vi "MStar Daily產能安排Report.vi"() -> ()   [LabVIEW 2012]
uses:
  <vilib>/Utility/NIReport.llb/NI_report.lvclass
  <vilib>/addons/database/Connection.llb/DB Tools Open Connec (Path).vi
  <vilib>/addons/database/Connection.llb/Conn Execute.vi
  <vilib>/addons/database/Recordset.llb/Rec Fetch Recordset Data (R).vi
  <vilib>/addons/database/Recordset.llb/Rec Destroy - Connection.vi
  <vilib>/Utility/NIReport.llb/Append Text Table to Report (wrap).vi
  <vilib>/addons/database/_DB Variant To Data/Database Variant To Data.xnode
  <vilib>/addons/database/NI_Database_API.lvlib
  <vilib>/Utility/NIReport.llb/Excel/NI_Excel.lvclass
panel:
  out "recordset data":variant[][](array[variant])
  out "appended array":string[](array[string])
  in  "Report Template":path=path "O:/Monitor/Report/MachineArrange.xls"
  out "error out 2":errorcluster
  in  "Table Control":string[][](table)
  out "error out 3":errorcluster
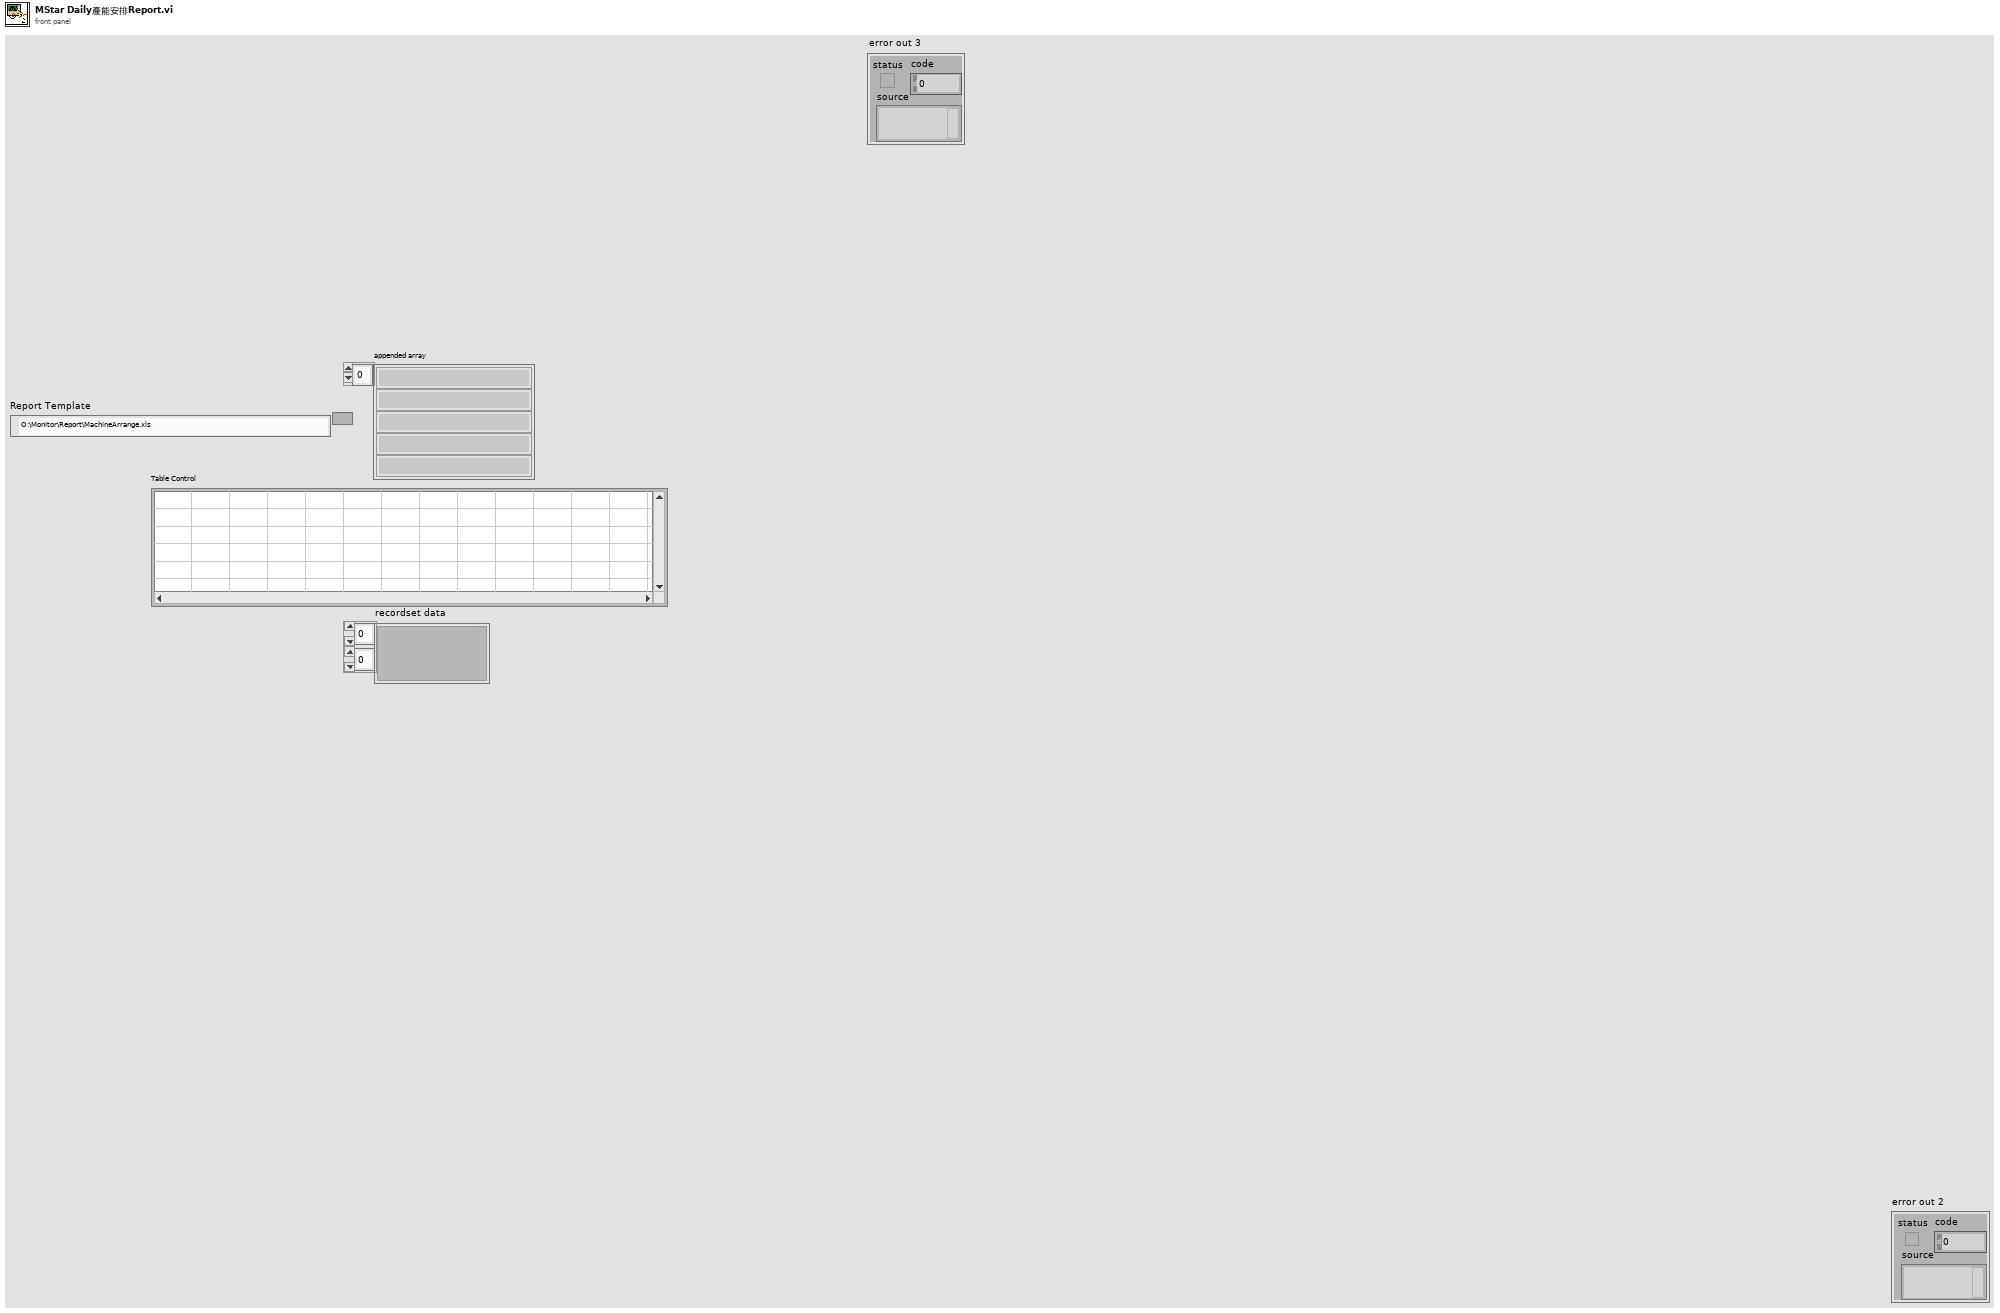
[diagram p1: front panel]
types:
  T1 = typedef "NI_Database_API.lvlib/Conn ObjectReference.ctl" = refnum<k1>
  T2 = typedef "NI_Database_API.lvlib/Rec ObjectReference.ctl" = refnum<k1>
  T3 = enum16{"Standard Report", "HTML", "Word", "Excel"}
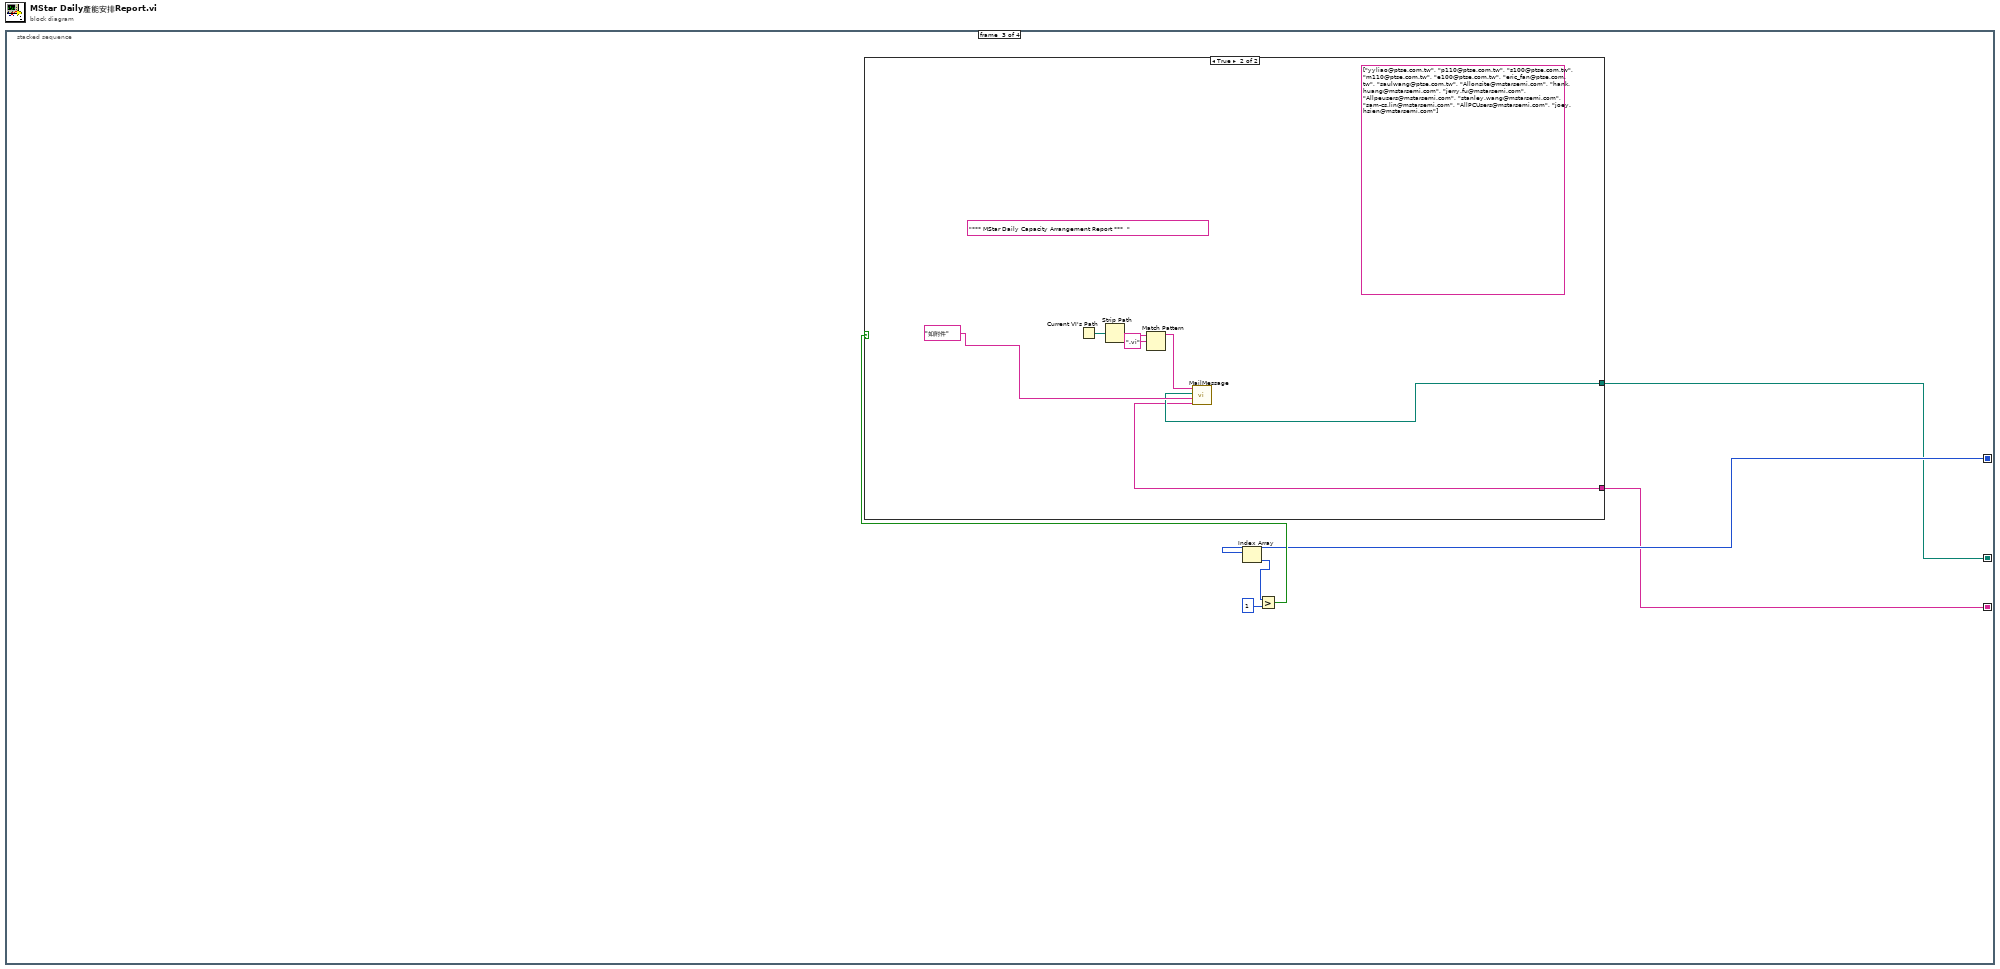
[diagram p0: block diagram]
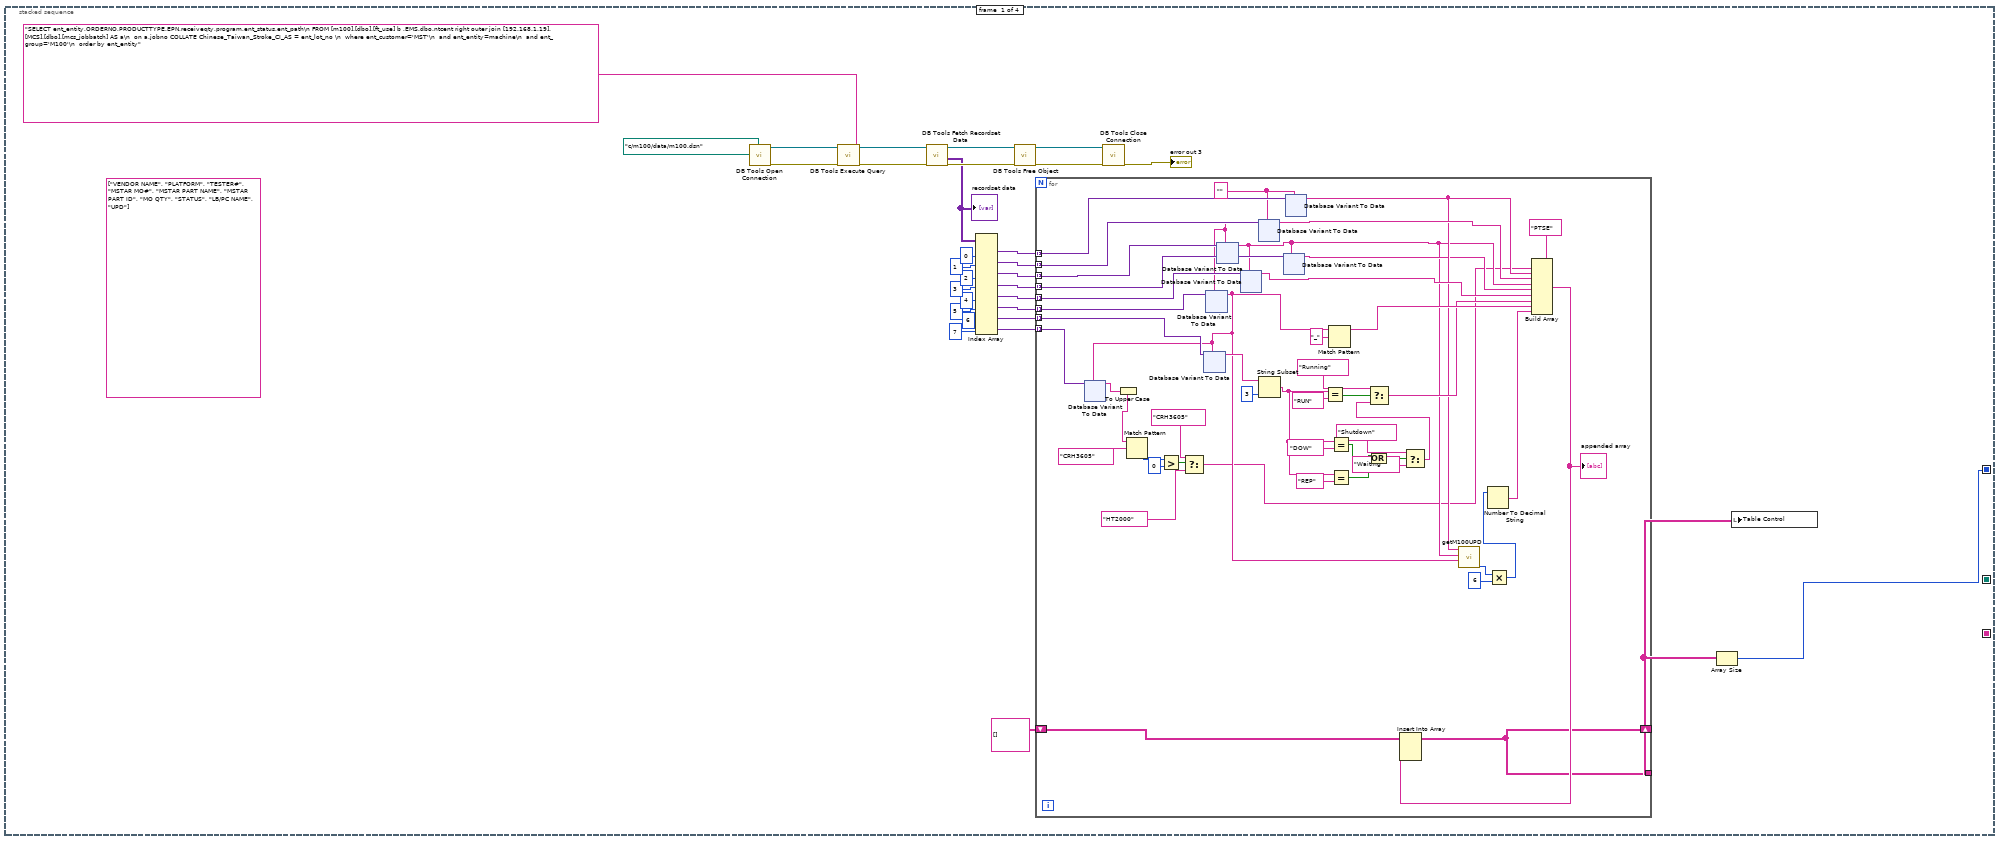
[diagram p2: hidden frame]
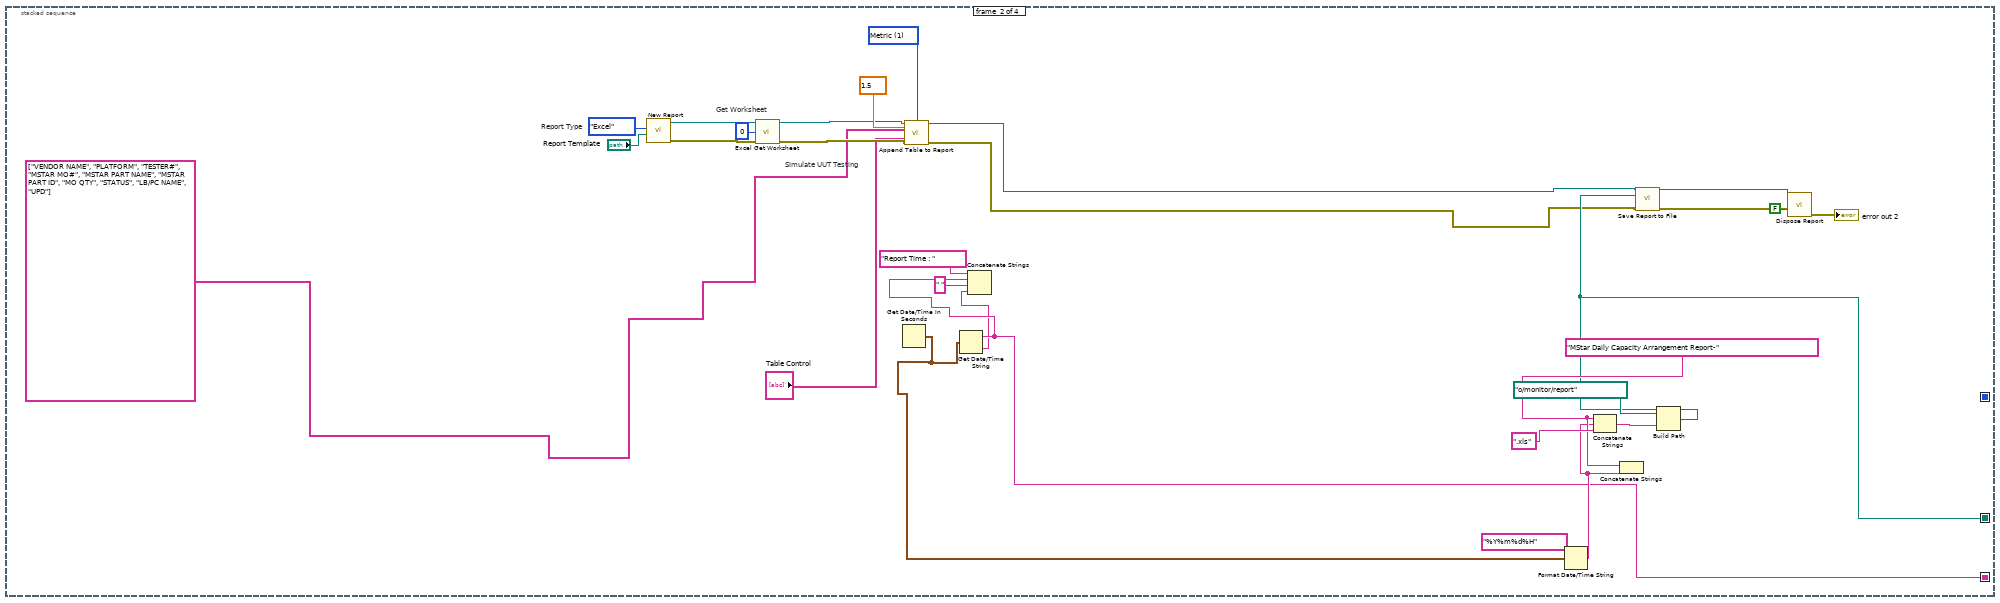
[diagram p3: hidden frame]
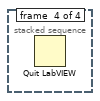
[diagram p5: hidden frame]
diagram:
  n1 = stacked-sequence {
    seq-local: [w5 _ _ _] -> [_ _ w368 _]
    seq-local: [_ w345 _ _] -> [_ _ w367 _]
    seq-local: [_ w342 _ _] -> [_ _ w366 _]
    frame #0 {
      (unwired) string[] ["VENDOR NAME", "PLATFORM", "TESTER#", "MSTAR MO#", "MSTAR PART NAME", "MSTAR PART ID", "MO QTY", "STATUS", "LB/PC NAME", "UPD"] ("row headers")
      n2 = call-poly <vilib>:"DB Tools Open Connection.vi"("connection information"=path "c:/m100/data/m100.dsn") -> ("error out"=w26:errorcluster, "connection reference"=w30:T1)  [unwired: 7 in]
      n3 = call-poly <vilib>:"DB Tools Execute Query.vi"("error in (no error)"=w26, "SQL query"="SELECT ent_entity,ORDERNO,PRODUCTTYPE,EPN,receiveqty,program,ent_status,ent_path\n FROM [m100].[dbo].[ft_use] b ,EMS.dbo.ntcent right outer join [192.168.1.19].[MCS].[dbo].[mcs_jobbatch] AS a\n  on a.jobno COLLATE Chinese_Taiwan_Stroke_CI_AS = ent_lot_no \n  where ent_customer='MST'\n  and ent_entity=machine\n  and ent_group='M100'\n  order by ent_entity", "connection reference"=w30) -> ("error out"=w25:errorcluster, "recordset reference"=w29:T2)  [unwired: 5 in]
      n4 = call-poly <vilib>:"DB Tools Fetch Recordset Data.vi"("error in (no error)"=w25, "recordset reference"=w29) -> ("error out"=w24:errorcluster, "recordset data"=w8:variant[][], "recordset reference out"=w28:T2)  [unwired: 3 in]
      "recordset data" <- w8
      n5 = Index Array(array=w8, index (col) #1=0 ("disabled index (col)"), index (col) #2=1 ("index (col)"), index (col) #3=2 ("index (col)"), index (col) #4=3 ("index (col)"), index (col) #5=4 ("index (col)"), index (col) #6=5 ("index (col)"), index (col) #7=6 ("index (col)"), index (col) #8=7 ("index (col)")) -> (element #1=w15:variant[], element #2=w14:variant[], element #3=w13:variant[], element #4=w12:variant[], element #5=w11:variant[], element #6=w10:variant[], element #7=w3:variant[], element #8=w1:variant[])  [unwired: 8 in]
      n6 = call-poly <vilib>:"DB Tools Free Object.vi"("error in (no error)"=w24, "recordset reference"=w28) -> ("error out"=w23:errorcluster, "connection reference"=w27:T1)  [unwired: 8 in]
      n7 = for {
        tunnel: w15 -> [w80] mode=indexing
        tunnel: w14 -> [w79] mode=indexing
        tunnel: w13 -> [w78] mode=indexing
        tunnel: w12 -> [w77] mode=indexing
        tunnel: w11 -> [w76] mode=indexing
        tunnel: w10 -> [w75] mode=indexing
        tunnel: [w73] -> w6
        shift-right: [w73] -> _
        shift-left: string[][] [] -> [w72]
        tunnel: w3 -> [w66] mode=indexing
        tunnel: w1 -> [w45] mode=indexing
        w70 = ""
        n8 = xnode "Database Variant To Data"("database variant"=w75, "type"=w70) -> ("data"=w44:string)  [unwired: 1 in, 1 out]
        n9 = xnode "Database Variant To Data"("database variant"=w45, "type"=w44) -> ("data"=w36:string)  [unwired: 1 in, 1 out]
        n10 = To Upper Case(1:w36) -> (0:w35:string)
        n11 = Match Pattern(string=w35, regular expression="CRH3605") -> (offset past match=w42:i32)  [unwired: 1 in, 3 out]
        n12 = Greater?(x=w42, y=0) -> (0:w40:bool)
        n13 = Select(t="CRH3605", s=w40, f="HT2000") -> (s? t:f=w37:string)
        n14 = xnode "Database Variant To Data"("database variant"=w66, "type"=w44) -> ("data"=w65:string)  [unwired: 1 in, 1 out]
        n15 = xnode "Database Variant To Data"("database variant"=w78, "type"=w70) -> ("data"=w46:string)  [unwired: 1 in, 1 out]
        n16 = xnode "Database Variant To Data"("database variant"=w76, "type"=w46) -> ("data"=w69:string)  [unwired: 1 in, 1 out]
        n17 = xnode "Database Variant To Data"("database variant"=w79, "type"=w70) -> ("data"=w71:string)  [unwired: 1 in, 1 out]
        n18 = String Subset(string=w65, length (rest)=3 ("length (rest)")) -> (substring=w58:string)  [unwired: 1 in]
        n19 = xnode "Database Variant To Data"("database variant"=w77, "type"=w46) -> ("data"=w48:string)  [unwired: 1 in, 1 out]
        n20 = xnode "Database Variant To Data"("database variant"=w80, "type"=w70) -> ("data"=w49:string)  [unwired: 1 in, 1 out]
        n21 = Equal?(x=w58, y="RUN") -> (x = y?=w62:bool)
        n22 = Match Pattern(string=w44, regular expression="_") -> (before substring=w51:string)  [unwired: 1 in, 3 out]
        n23 = Equal?(x=w58, y="DOW") -> (x = y?=w57:bool)
        n24 = Equal?(x=w58, y="REP") -> (x = y?=w56:bool)
        n25 = Or(x=w57, y=w56) -> (x .or. y?=w55:bool)
        n26 = Select(t="Shutdown" ("y"), s=w55, f="Waiting") -> (s? t:f=w52:string)
        n27 = Select(t="Running" ("y"), s=w62, f=w52) -> (s? t:f=w50:string)
        n28 = call "getM100UPD.vi"("Program"=w44, "Product"=w46, "Machine"=w49) -> ("UPD"=w34:i32)  [unwired: 5 in, 3 out]
        n29 = Multiply(x=w34, y=6) -> (x*y=w32:i32)
        n30 = Number To Decimal String(number=w32) -> (decimal integer string=w47:string)  [unwired: 1 in]
        n31 = Build Array("PTSE", w37, w49, w71, w46, w48, w69, w50, w51, w47) -> (w74:string[])
        "appended array" <- w74
        n32 = Insert Into Array(array=w72, new element=w74) -> (w73:string[][])  [unwired: 2 in]
      }
      n33 = call <vilib>:"DB Tools Close Connection.vi"("error in (no error)"=w23, "connection reference"=w27) -> ("error out"=→"error out 3":errorcluster)  [unwired: 5 in]
      n34 = Array Size(array=w6) -> (size(s)=w5:i32[])
      n35 = local write "Table Control"(w6) -> ()
    }
    frame #1 {
      w349 = u16 1 items=["US", "Metric", "Default"] ("measurement system")
      w350 = "MStar Daily Capacity Arrangement Report-"
      w365 = T3."Excel"  # Report Type
      # "Simulate UUT Testing"
      # "Get Worksheet"
      n36 = call <vilib>:"New Report.vi"("report type"=w365, "template (empty)"="Report Template") -> ("report out"=w362:refnum<class "NI_report.lvclass">, "error out"=w361:errorcluster)  [unwired: 12 in]
      n37 = call <vilib>:"Excel Get Worksheet.vi"("report in"=w362, "worksheet index (0)"=0, "error in (no error)"=w361) -> ("report out"=w355:refnum<class "NI_report.lvclass">, "error out"=w354:errorcluster)  [unwired: 11 in]
      n38 = Get Date/Time In Seconds() -> (seconds since 1Jan1904=w340:timestamp)
      n39 = call-poly <vilib>:"Append Table to Report.vi"("report in"=w355, "column width (1)"=1.5, "measurement system"=w349, "column headers"=string[] ["VENDOR NAME", "PLATFORM", "TESTER#", "MSTAR MO#", "MSTAR PART NAME", "MSTAR PART ID", "MO QTY", "STATUS", "LB/PC NAME", "UPD"] ("row headers"), "text data"="Table Control", "error in (no error)"=w354) -> ("report out"=w338:refnum<class "NI_report.lvclass">, "error out"=w337:errorcluster)  [unwired: 6 in, 2 out]
      n40 = Get Date/Time String(seconds (now)=w340) -> (date string=w342:string, time string=w341:string)  [unwired: 2 in]
      n41 = Concatenate Strings("Report Time : " ("string"), w342, " " ("string"), w341) -> ()  [unwired: 1 out]
      n42 = Format Date/Time String(time format string (%c)="%Y%m%d%H", seconds (now)=w340) -> (date/time string=w347:string)  [unwired: 1 in]
      n43 = Concatenate Strings(w350, w347, ".xls" ("string")) -> (w351:string)
      n44 = Concatenate Strings(w350, w347) -> ()  [unwired: 1 out]
      n45 = Build Path(base path=path "o:/monitor/report", name or relative path=w351) -> (appended path=w345:path)
      n46 = call-dynamic "Save Report to File.vi"("report in"=w338, "report file path"=w345, "error in (no error)"=w337) -> ("report out"=w357:refnum<class "NI_report.lvclass">, "error out"=w356:errorcluster)  [unwired: 11 in]
      n47 = call-dynamic "Dispose Report.vi"("report in"=w357, "save changes? (F)"=FALSE, "error in (no error)"=w356) -> ("error out"=→"error out 2":errorcluster)  [unwired: 12 in]
    }
    frame #2 {
      n48 = Index Array(array=w368) -> (element=w371:i32)  [unwired: 1 in]
      n49 = Greater?(x=w371, y=1) -> (0:w369:bool)
      n50 = case shown="True" w369 {
        tunnel: w367 -> [_ w373]
        tunnel: w366 -> [_ w372]
        frame False {
        }
        frame True {
          (unwired) string[] ["yyliao@ptse.com.tw", "p110@ptse.com.tw", "s100@ptse.com.tw", "m110@ptse.com.tw", "e100@ptse.com.tw", "eric_fan@ptse.com.tw", "saulwang@ptse.com.tw", "Allonsite@mstarsemi.com", "hank.huang@mstarsemi.com", "jerry.fu@mstarsemi.com", "Allpeusers@mstarsemi.com", "stanley.wang@mstarsemi.com", "sam-cs.lin@mstarsemi.com", "AllPCUsers@mstarsemi.com", "joey.hsien@mstarsemi.com"] ("recipients")
          (unwired) "*** MStar Daily Capacity Arrangement Report ***  " ("subject ([No Subject])")
          n51 = Current VI's Path() -> (path=w378:path)
          n52 = Strip Path(path=w378) -> (name=w377:string)  [unwired: 1 out]
          n53 = Match Pattern(string=w377, regular expression=".vi") -> (before substring=w375:string)  [unwired: 1 in, 3 out]
          n54 = call "MailMessage.vi"("AddSubject"=w372, "message"="如附件", "file path"=w373, "program"=w375) -> ()  [unwired: 8 in]
        }
      }
    }
    frame #3 {
      n55 = Quit LabVIEW() -> ()  [unwired: 1 in]
    }
  }
